vi "Keyboard Input.vi"(0 "Loop Delay (ms)":dbl=10.0, 1 "Scaling Factor":dbl) -> (2 "Horizontal Output":dbl, 3 "Vertical Output":dbl, 4 "Key Output":dbl)   [LabVIEW 2012]
uses:
  <vilib>/Utility/inputDevices.llb/closeKeyboard.vi
  <vilib>/Utility/inputDevices.llb/keyboardAcquire.vi
panel:
  out "Key Output 2":dbl
  out "Vertical Output 2":dbl
  out "Horizontal Output 2":dbl
  out "Key Code String 2":string
  out "Key code 2":i32[](array[numeric])
  out "Running":bool
  out "Key Code String":string
  out "Key code":i32[](array[numeric])
  out "keys pressed":T1(array[ring])
  in  "stop":bool
  # "Left = 68\nRight = 92\nUp = 102\nDown = 59\nEnter = 91\nEscape = 62"
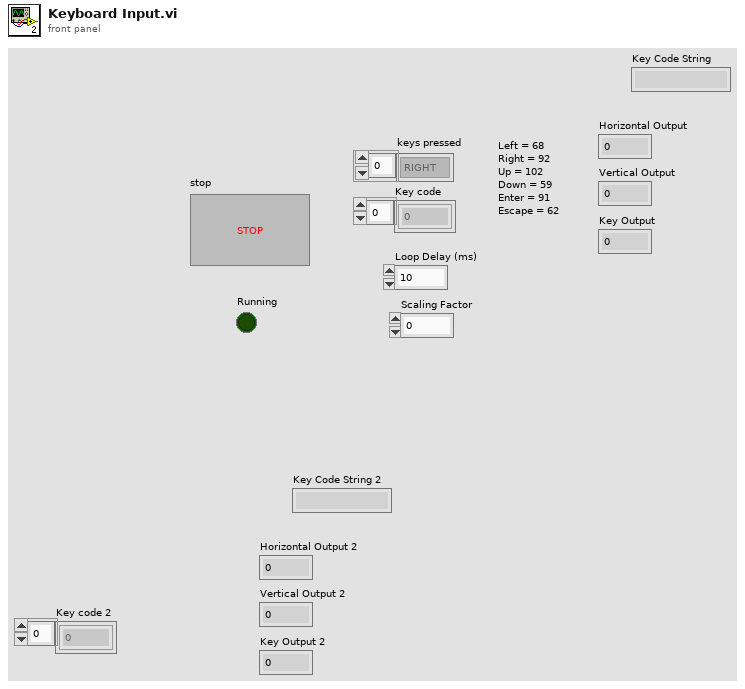
[diagram p1: front panel]
types:
  T1 = enum16{"0", "1", "2", "3", "4", "5", "6", "7", "8", "9", "A", "B", "C", "D", "E", "F", "G", "H", "I", "J", "K", "L", "M", "N", "O", "P", "Q", "R", "S", "T", "U", "V", "W", "X", "Y", "Z", "F1", "F2", "F3", "F4", "F5", "F6", "F7", "F8", "F9", "F10", "F11", "F12", "F13", "F14", "F15", "ADD", "BACK", "BACKSLASH", "CAPITAL", "COMMA", "DECIMAL", "DELETE", "DIVIDE", "DOWN", "END", "EQUALS", "ESCAPE", "GRAVE (`)", "HOME", "INSERT", "LBRACKET", "LCONTROL", "LEFT", "L ALT", "LSHIFT", "LWIN", "MINUS", "MULTIPLY", "NEXT", "NUMLOCK", "NUMPAD_0", "NUMPAD_1", "NUMPAD_2", "NUMPAD_3", "NUMPAD_4", "NUMPAD_5", "NUMPAD_6", "NUMPAD_7", "NUMPAD_8", "NUMPAD_9", "PAUSE", "PERIOD", "PRIOR (PG UP)", "RBRACKET", "RCONTROL", "RETURN", "RIGHT", "R ALT", "RSHIFT", "RWIN", "SCROLL", "SEMICOLON", "SLASH", "SPACE", "SUBTRACT", "TAB", "UP", "ENTER (num pad)", "' (quote)"}[]
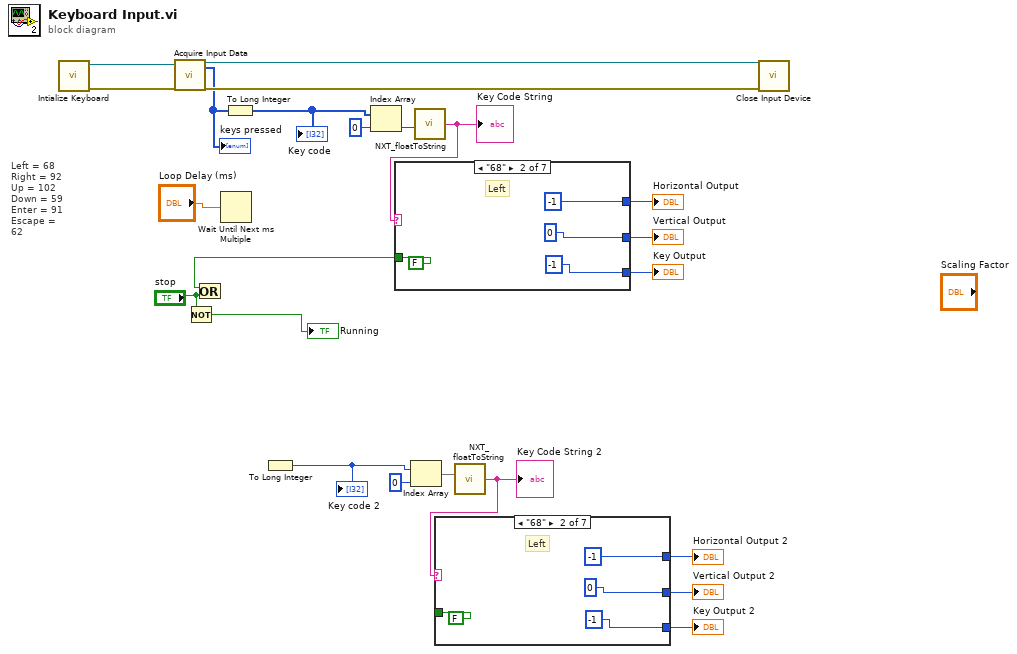
[diagram p0: block diagram]
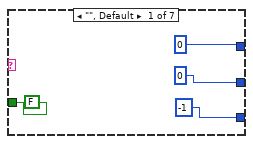
[diagram p2: hidden frame]
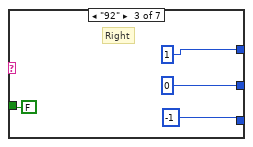
[diagram p3: hidden frame]
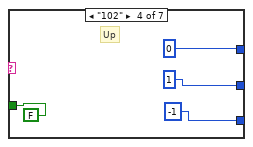
[diagram p4: hidden frame]
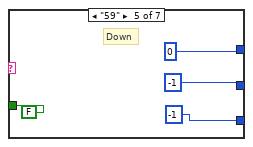
[diagram p5: hidden frame]
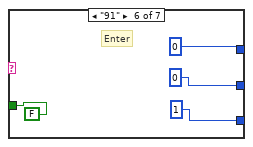
[diagram p6: hidden frame]
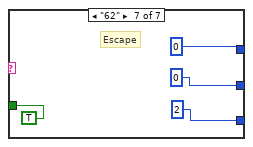
[diagram p7: hidden frame]
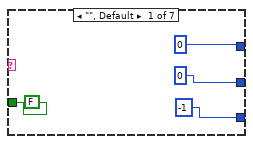
[diagram p8: hidden frame]
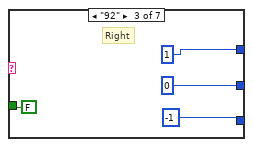
[diagram p9: hidden frame]
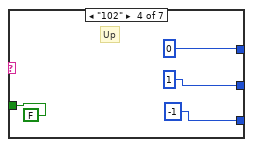
[diagram p10: hidden frame]
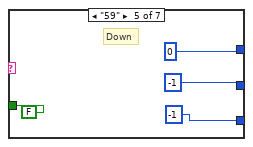
[diagram p11: hidden frame]
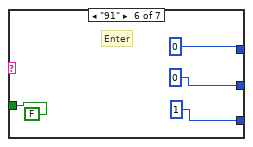
[diagram p12: hidden frame]
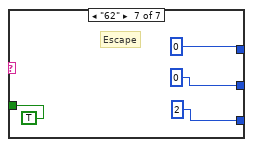
[diagram p13: hidden frame]
diagram:
  # "Left = 68\nRight = 92\nUp = 102\nDown = 59\nEnter = 91\nEscape = 62"
  n1 = call <vilib>:"Intialize Keyboard.vi"() -> ("error out"=w22:errorcluster, "device ID"=w23:refnum<k1>)  [unwired: 10 in]
  n2 = call-poly <vilib>:"Acquire Input Data.vi"("device ID"=w23, "error in (no error)"=w22) -> ("device ID"=w21:refnum<k1>, "keys pressed"=w19:T1, "error out"=w20:errorcluster)  [unwired: 15 in]
  "keys pressed" <- w19
  n3 = Not(x="stop") -> (.not. x?=→"Running":bool)
  n4 = Wait Until Next ms Multiple(millisecond multiple="Loop Delay (ms)") -> ()  [unwired: 1 out]
  n5 = To Long Integer(number=w19) -> (32bit integer=w17:i32[])
  "Key code" <- w17
  n6 = To Long Integer() -> (32bit integer=w7:i32)  [unwired: 1 in]
  "Key code 2" <- w7
  n7 = Index Array(array=w17, index=0) -> (element=w15:i32)
  n8 = Index Array(array=w7, index=0) -> (element=w5)
  n9 = call <vilib>:"NXT_floatToString.vi"("number"=w15) -> ("string"=w14:string)
  "Key Code String" <- w14
  n10 = case shown="\"68\"" w14 {
    tunnel: [FALSE FALSE FALSE FALSE FALSE FALSE TRUE] -> w12
    tunnel: [0 -1 1 0 0 0 0] -> w11
    tunnel: [0 0 0 1 -1 0 0] -> w10
    tunnel: [-1 -1 -1 -1 -1 1 2] -> w9
    frame "", Default {
    }
    frame "68" {
      # "Left"
    }
    frame "92" {
      # "Right"
    }
    frame "102" {
      # "Up"
    }
    frame "59" {
      # "Down"
    }
    frame "91" {
      # "Enter"
    }
    frame "62" {
      # "Escape"
    }
  }
  "Horizontal Output" <- w11
  "Vertical Output" <- w10
  "Key Output" <- w9
  n11 = Or(x=w12, y="stop") -> ()  [unwired: 1 out]
  n12 = call <vilib>:"NXT_floatToString.vi"("number"=w5) -> ("string"=w4:string)
  "Key Code String 2" <- w4
  n13 = case shown="\"68\"" w4 {
    tunnel: [FALSE FALSE FALSE FALSE FALSE FALSE TRUE] -> _
    tunnel: [0 -1 1 0 0 0 0] -> w3
    tunnel: [0 0 0 1 -1 0 0] -> w2
    tunnel: [-1 -1 -1 -1 -1 1 2] -> w1
    frame "", Default {
    }
    frame "68" {
      # "Left"
    }
    frame "92" {
      # "Right"
    }
    frame "102" {
      # "Up"
    }
    frame "59" {
      # "Down"
    }
    frame "91" {
      # "Enter"
    }
    frame "62" {
      # "Escape"
    }
  }
  "Horizontal Output 2" <- w3
  "Vertical Output 2" <- w2
  "Key Output 2" <- w1
  n14 = call-poly <vilib>:"Close Input Device.vi"("error in (no error)"=w20, "device ID"=w21) -> ()  [unwired: 8 in, 1 out]
